vi "get_EQgroup.vi"(9 "Process":string, 11 "Package":string) -> (2 "EQ Grp":string)   [LabVIEW 2012]
uses:
  <vilib>/addons/database/Connection.llb/DB Tools Open Connec (Path).vi
  <vilib>/addons/database/Connection.llb/Conn Execute.vi
  <vilib>/addons/database/Recordset.llb/Rec Fetch String Data (R).vi
  <vilib>/addons/database/Recordset.llb/Rec Destroy - Connection.vi
  <vilib>/addons/database/NI_Database_API.lvlib
panel:
  out "error out":errorcluster
  out "concatenated string":string
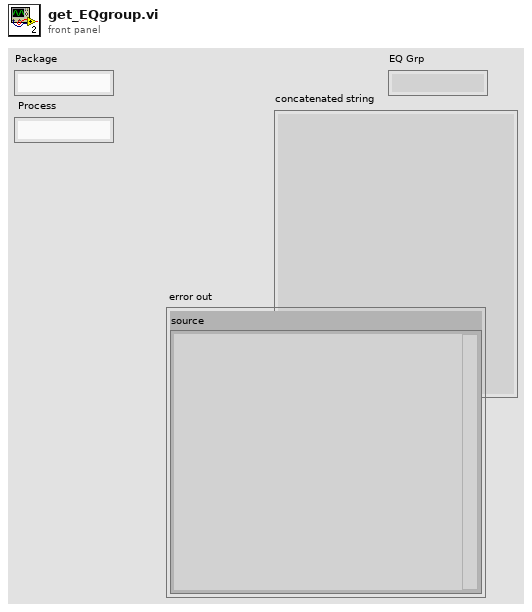
[diagram p1: front panel]
types:
  T1 = typedef "NI_Database_API.lvlib/Conn ObjectReference.ctl" = refnum<k1>
  T2 = typedef "NI_Database_API.lvlib/Rec ObjectReference.ctl" = refnum<k1>
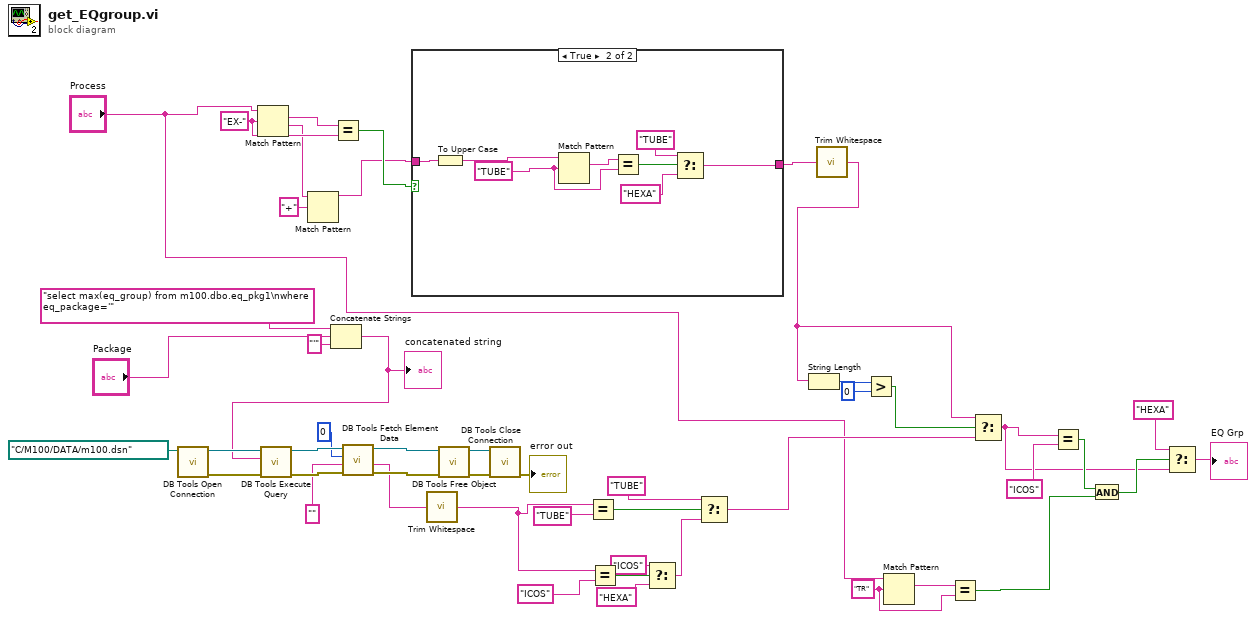
[diagram p0: block diagram]
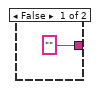
[diagram p2: hidden frame]
diagram:
  w8 = "TR" ("regular expression")
  w47 = "EX-" ("regular expression")
  n1 = call-poly <vilib>:"DB Tools Open Connection.vi"("connection information"=path "C:/M100/DATA/m100.dsn") -> ("error out"=w38:errorcluster, "connection reference"=w39:T1)  [unwired: 7 in]
  n2 = Match Pattern(string="Process", regular expression=w47) -> (match substring=w48:string, after substring=w18:string)  [unwired: 1 in, 2 out]
  n3 = Match Pattern(string=w18, regular expression="+") -> (before substring=w16:string)  [unwired: 1 in, 3 out]
  n4 = Concatenate Strings("select max(eq_group) from m100.dbo.eq_pkg1\nwhere eq_package='" ("string"), "Package", "'" ("string")) -> (w33:string)
  "concatenated string" <- w33
  n5 = call-poly <vilib>:"DB Tools Execute Query.vi"("error in (no error)"=w38, "SQL query"=w33, "connection reference"=w39) -> ("error out"=w40:errorcluster, "recordset reference"=w41:T2)  [unwired: 5 in]
  n6 = Equal?(x=w48, y=w47) -> (x = y?=w46:bool)
  n7 = call-poly <vilib>:"DB Tools Fetch Element Data.vi"("error in (no error)"=w40, "type"="", "column index"=0, "recordset reference"=w41) -> ("error out"=w42:errorcluster, "data"=w13:string, "recordset reference out"=w43:T2)  [unwired: 3 in]
  n8 = case shown="True" w46 {
    tunnel: w16 -> [_ w57]
    tunnel: ["" ("f") w50] -> w15
    frame False {
    }
    frame True {
      w55 = "TUBE" ("regular expression")
      n9 = To Upper Case(1:w57) -> (0:w52:string)
      n10 = Match Pattern(string=w52, regular expression=w55) -> (match substring=w56:string)  [unwired: 1 in, 3 out]
      n11 = Equal?(x=w56, y=w55) -> (x = y?=w54:bool)
      n12 = Select(t="TUBE", s=w54, f="HEXA") -> (s? t:f=w50:string)
    }
  }
  n13 = call <vilib>:"Trim Whitespace.vi"("string"=w13) -> ("trimmed string"=w12:string)  [unwired: 1 in]
  n14 = call-poly <vilib>:"DB Tools Free Object.vi"("error in (no error)"=w42, "recordset reference"=w43) -> ("error out"=w45:errorcluster, "connection reference"=w44:T1)  [unwired: 8 in]
  n15 = call <vilib>:"DB Tools Close Connection.vi"("error in (no error)"=w45, "connection reference"=w44) -> ("error out"=→"error out":errorcluster)  [unwired: 5 in]
  n16 = Equal?(x=w12, y="TUBE") -> (x = y?=w30:bool)
  n17 = Equal?(x=w12, y="ICOS") -> (x = y?=w28:bool)
  n18 = Select(t="ICOS", s=w28, f="HEXA") -> (s? t:f=w25:string)
  n19 = Select(t="TUBE", s=w30, f=w25) -> (s? t:f=w21:string)
  n20 = call <vilib>:"Trim Whitespace.vi"("string"=w15) -> ("trimmed string"=w14:string)  [unwired: 1 in]
  n21 = String Length(string=w14) -> (length=w24:i32)
  n22 = Greater?(x=w24, y=0) -> (0:w22:bool)
  n23 = Match Pattern(string="Process", regular expression=w8) -> (match substring=w9:string)  [unwired: 1 in, 3 out]
  n24 = Equal?(x=w9, y=w8) -> (x = y?=w5:bool)
  n25 = Select(t=w14, s=w22, f=w21) -> (s? t:f=w3:string)
  n26 = Equal?(x=w3, y="ICOS") -> (x = y?=w6:bool)
  n27 = And(x=w6, y=w5) -> (x .and. y?=w4:bool)
  n28 = Select(t="HEXA", s=w4, f=w3) -> (s? t:f=→"EQ Grp":string)
